vi "COD浓度全局变量.vi"() -> ()   [LabVIEW 2016, in "斯坦道CODMn.lvlib"]
uses:
  <vilib>/Plasmionique/MB Master/MB_Master_Serial/MB_Master_Serial.lvclass
panel:
  in  "Error in":errorcluster
  in  "MB_Serial session":refnum<class "MB_Master_Serial.lvclass">
  in  "VISA resource name":refnum<visa-resource-name>="COM4" caption="VISA资源名称"
  in  "基本量程":enum16{"10mg/L", "20mg/L"}(ring)
  in  "浓度 2":dbl
  in  "跨度液浓度":dbl
  in  "COD浓度（mg/L)":dbl
  # "跨度液浓度："
  # "标准液浓度（mg/L）："
  # "基本量程（20mL可选）："
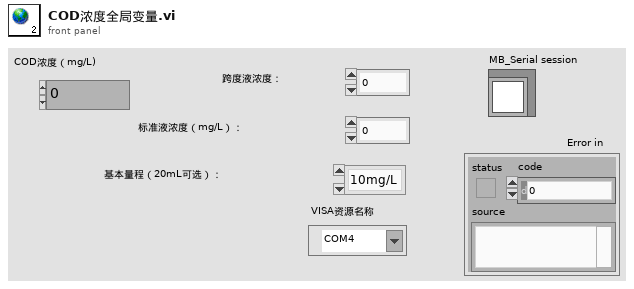
[diagram p1: front panel]
diagram:
